vi "RTTTL_Note_Parse.vi"(3 "Element":string, 4 "Beat":dbl, 5 "Default octave":dbl, 6 "Default duration":dbl) -> (0 "Pause":dbl, 1 "Duration":dbl, 2 "Frequency":i32)   [LabVIEW 2011]
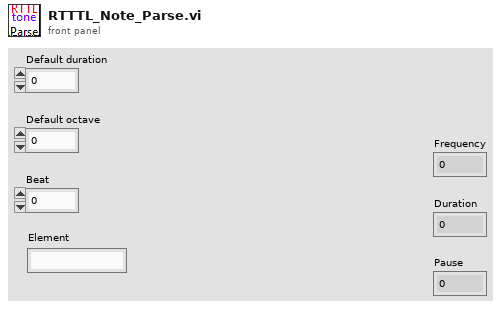
[diagram p1: front panel]
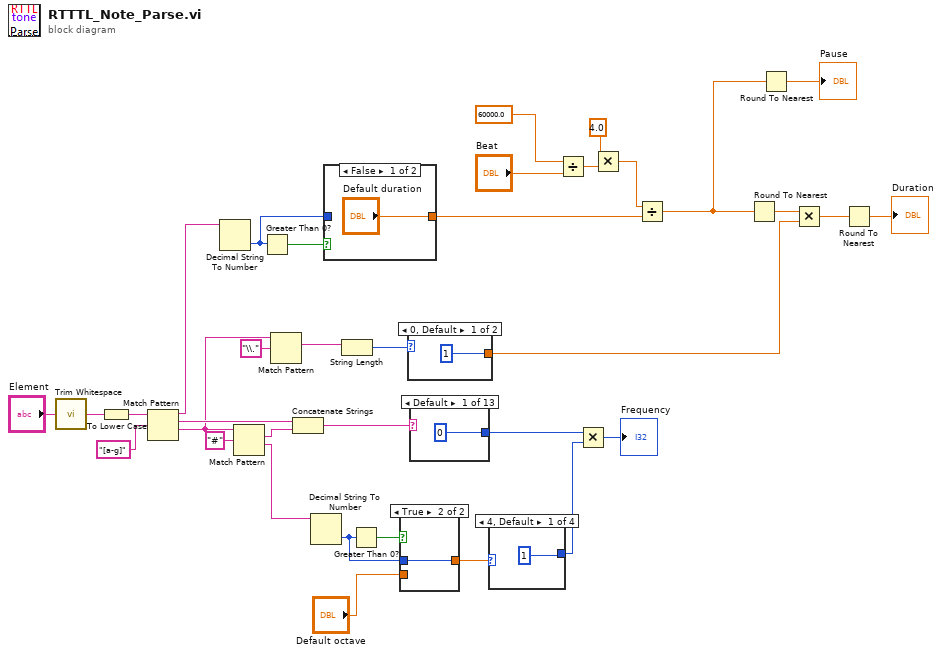
[diagram p0: block diagram]
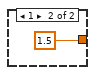
[diagram p2: hidden frame]
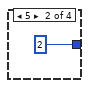
[diagram p3: hidden frame]
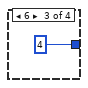
[diagram p4: hidden frame]
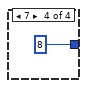
[diagram p5: hidden frame]
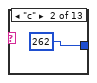
[diagram p8: hidden frame]
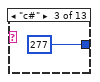
[diagram p9: hidden frame]
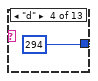
[diagram p10: hidden frame]
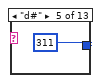
[diagram p11: hidden frame]
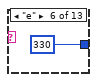
[diagram p12: hidden frame]
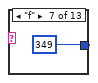
[diagram p13: hidden frame]
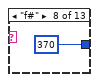
[diagram p14: hidden frame]
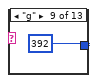
[diagram p15: hidden frame]
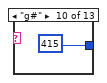
[diagram p16: hidden frame]
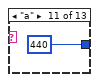
[diagram p17: hidden frame]
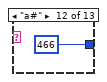
[diagram p18: hidden frame]
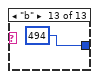
[diagram p19: hidden frame]
diagram:
  n1 = call <vilib>:"Trim Whitespace.vi"("string"="Element") -> ("trimmed string"=w33:string)  [unwired: 1 in]
  n2 = To Lower Case(string=w33) -> (all lower case string=w31:string)
  n3 = Match Pattern(string=w31, regular expression="[a-g]") -> (before substring=w27:string, match substring=w30:string, after substring=w7:string)  [unwired: 1 in, 1 out]
  n4 = Decimal String To Number(string=w27) -> (number=w24:i32)  [unwired: 2 in, 1 out]
  n5 = Match Pattern(string=w7, regular expression="#") -> (match substring=w29:string, after substring=w26:string)  [unwired: 1 in, 2 out]
  n6 = Greater Than 0?(x=w24) -> (x > 0?=w25:bool)
  n7 = Match Pattern(string=w7, regular expression="\\.") -> (match substring=w6:string)  [unwired: 1 in, 3 out]
  n8 = Concatenate Strings(w30, w29) -> (w28:string)
  n9 = Decimal String To Number(string=w26) -> (number=w22:i32)  [unwired: 2 in, 1 out]
  n10 = case shown="False" w25 {
    tunnel: w24 -> [_ w37]
    tunnel: ["Default duration" w37] -> w12
    frame False {
    }
    frame True {
    }
  }
  n11 = String Length(string=w6) -> (length=w5:i32)
  n12 = Greater Than 0?(x=w22) -> (x > 0?=w23:bool)
  n13 = case shown="True" w23 {
    tunnel: w22 -> [_ w39]
    tunnel: [w38 w39] -> w19
    tunnel: "Default octave" -> [w38 _]
    frame False {
    }
    frame True {
    }
  }
  n14 = case shown="0, Default" w5 {
    tunnel: [1 1.5] -> w4
    frame 0, Default {
    }
    frame 1 {
    }
  }
  n15 = case shown="Default" w28 {
    tunnel: [0 262 277 294 311 330 349 370 392 415 440 466 494] -> w20
    frame Default {
    }
    frame "c" {
    }
    frame "c#" {
    }
    frame "d" {
    }
    frame "d#" {
    }
    frame "e" {
    }
    frame "f" {
    }
    frame "f#" {
    }
    frame "g" {
    }
    frame "g#" {
    }
    frame "a" {
    }
    frame "a#" {
    }
    frame "b" {
    }
  }
  n16 = case shown="4, Default" w19 {
    tunnel: [1 2 4 8] -> w18
    frame 4, Default {
    }
    frame 5 {
    }
    frame 6 {
    }
    frame 7 {
    }
  }
  n17 = Divide(x=60000.0, y="Beat") -> (x/y=w13:dbl)
  n18 = Multiply(x=w20, y=w18) -> (x*y=→"Frequency":i32)
  n19 = Multiply(x=4.0, y=w13) -> (x*y=w11:dbl)
  n20 = Divide(x=w11, y=w12) -> (x/y=w9:dbl)
  n21 = Round To Nearest(number=w9) -> (nearest integer value=w3:dbl)
  n22 = Round To Nearest(number=w9) -> (nearest integer value=→"Pause":dbl)
  n23 = Multiply(x=w3, y=w4) -> (x*y=w1:dbl)
  n24 = Round To Nearest(number=w1) -> (nearest integer value=→"Duration":dbl)
